vi "Actor Core.vi"(8 "error in":errorcluster, 11 "IMAQ Display in":refnum<class "HIJ Vision Display.lvclass">) -> (0 "error out":errorcluster, 3 "Actor out":refnum<class "Actor.lvclass">)   [LabVIEW 2020, in "HIJ Vision Display.lvlib" / "HIJ Vision Display.lvclass"]
doc: "(<B>Filename</B>: Actor Framework.lvlib:Actor.lvclass:Actor Core.vi)\n\nReceives messages to the actor, reacts to them, and initiates any error handling that may shut the actor down.\n\nDescendant classes may override this VI to append parallel tasks for the actor to complete while it handles messages. Overrides use the Call Parent Method node."
uses:
  HIJ Vision Display.lvclass
  C:/Users/AlexK/work/LabVIEW Programme/POLARIS CAM Log Abw und E/Submodules/Viewable Actor/ViewableActor/ViewableActor.lvclass
  C:/Program Files (x86)/National Instruments/LabVIEW 2020/vi.lib/ActorFramework/Actor/Actor.lvclass
  <vilib>/ActorFramework/Actor/Actor.lvclass
  Palette.ctl
  HIJ Vision Display.lvclass/HIJ Vision Display.ctl
  <vilib>/ActorFramework/Actor/Actor.lvclass/Actor.ctl
  <vilib>/ActorFramework/Message Enqueuer/Message Enqueuer.lvclass/Message Enqueuer.ctl
  HIJ Vision Display Messages/Write ROI Msg/Write ROI Msg.lvclass/Write ROI Msg.ctl
  HIJ Vision Display Messages/Mouse Click Coords Msg/Mouse Click Coords Msg.lvclass/Mouse Click Coords Msg.ctl
  HIJ Vision Display Messages/Send Reply Actor State/Send Reply Actor State.lvclass
  C:/Program Files (x86)/National Instruments/LabVIEW 2020/vi.lib/ActorFramework/Reply Msg/Reply Msg.lvclass
  <vilib>/ActorFramework/Message Enqueuer/Message Priority.ctl
  <vilib>/ActorFramework/Reply Msg/Reply Msg.lvclass/Reply Msg.ctl
  HIJ Vision Display Messages/Contex Menu Selection Msg/Contex Menu Selection Msg.lvclass/Contex Menu Selection Msg.ctl
  <vilib>/ActorFramework/Message Enqueuer/Init from Existing Queue.vi
  <vilib>/ActorFramework/Message Enqueuer/Enqueue.vi
  HIJ Vision Display Messages/Write ROI Msg/Write ROI Msg.lvclass
  C:/Program Files (x86)/National Instruments/LabVIEW 2020/vi.lib/ActorFramework/Message/Message.lvclass
  HIJ Vision Display Messages/Evaluate with new Params Msg/Evaluate with new Params Msg.lvclass
  HIJ Vision Display Messages/Mouse Click Coords Msg/Mouse Click Coords Msg.lvclass
  <vilib>/ActorFramework/Reply Msg/Reply Msg.lvclass
  HIJ Vision Display Messages/Contex Menu Selection Msg/Contex Menu Selection Msg.lvclass
  HIJ Vision Display Messages/Show or Hide QSettings Msg/Show or Hide QSettings Msg.lvclass
  <vilib>/ActorFramework/Message Priority Queue/Priority Enqueue.vi
  <vilib>/ActorFramework/Message Enqueuer/Message Enqueuer.lvclass
  Viewable Actor/ViewableActor/ViewableActor.lvclass
  Utility/POLARIS Vision utility.lvlib
  C:/Users/AlexK/work/LabVIEW Programme/POLARIS CAM Log Abw und E/Submodules/HIJ Vision/Display Actors/HIJ Vision Display/HIJ Vision Display Messages/Send Reply Actor State/Send Reply Actor State.lvclass
panel:
  out "Acq Stoped Ind":bool caption="Acquistion stoped!"
  in  "Zoom Buttons":T1(radio)
  out "Image":T2(plugin-control)
  in  "StopSignal":bool=TRUE
  in  "Pallete":T3={"Teiler"=1, "Palette Type"=2} {"Teiler" min=1 max=5; "Palette Type" items=["Grayscale", "Binary", "Gradient", "Rainbow", "Temperature", "User Defined"]}
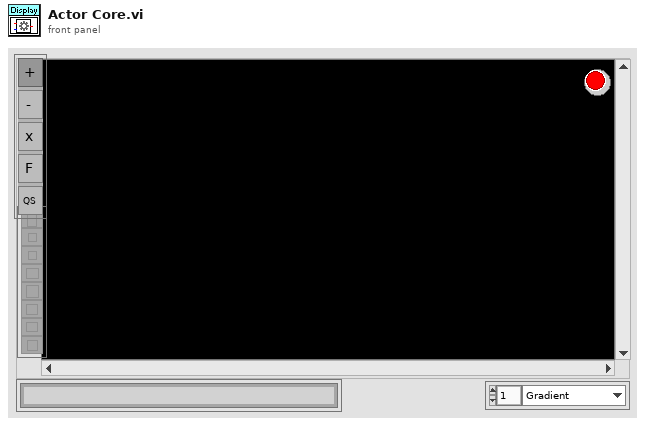
[diagram p1: front panel]
types:
  T1 = enum32{"Zoom in", "Zoom out", "Center", "Zoom to Fit", "Show Quick Settings"}
  T2 = typedef "IMAQ Image.ctl" = refnum<image>
  T3 = typedef "HIJ Vision Display.lvlib/HIJ Vision Display.lvclass/Palette.ctl" = cluster{"Teiler":i32, "Palette Type":u32}
  T4 = enum32{"Zoom in", "Zoom out", "Center", "Zoom to Fit"}
  T5 = cluster{"Zoom Tool":bool, "Selection Tool":bool, "Pan Tool":bool, "Point Tool":bool, "Line Tool":bool, "Rectangle Tool":bool, "Rotated Rectangle Tool":bool, "Polyline Tool":bool, "Polygon Tool":bool, "Freehand Tool":bool, "Closed Freehand Tool":bool, "Ellipse Tool":bool, "Annulus Tool":bool}
  T6 = typedef "Actor Framework.lvlib/Message Enqueuer.lvclass/Message Priority.ctl" = enum16{"Low", "Normal", "High"}
  T7 = cluster{"Global Rectangle":i32[], "Contours":cluster{"Contour Type":u32, "ROI Type":u32, "Points":i32[]}[]}
  T8 = typedef "LVPositionTypeDef.ctl" = cluster{"Left":i32, "Top":i32}
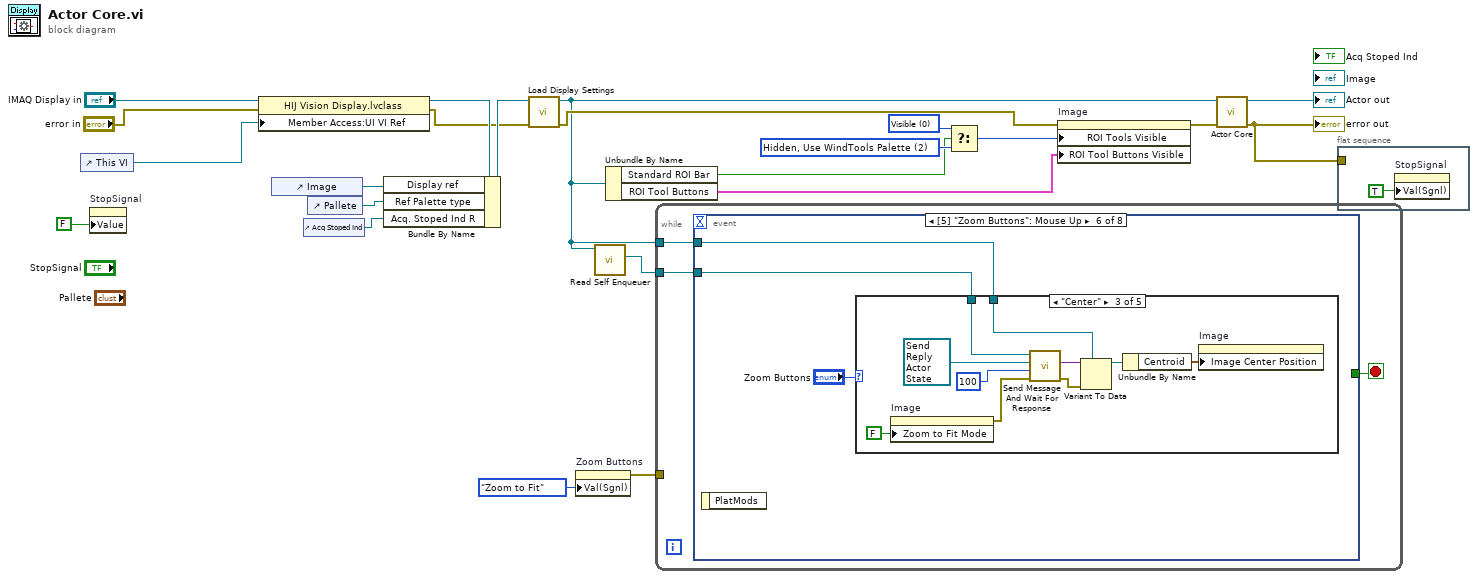
[diagram p0: block diagram]
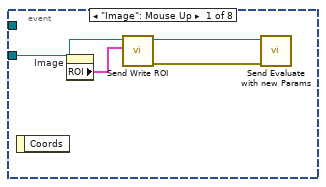
[diagram p2: hidden frame]
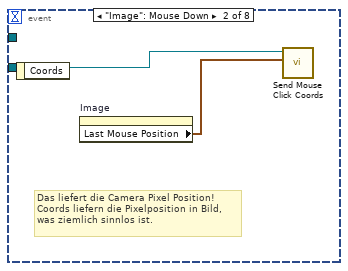
[diagram p3: hidden frame]
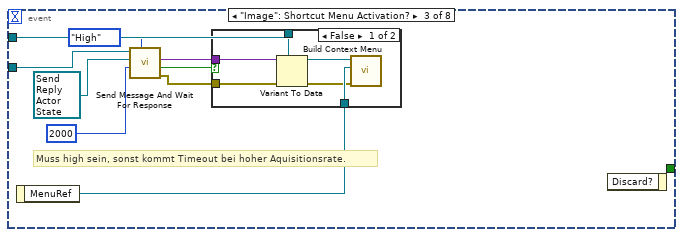
[diagram p4: hidden frame]
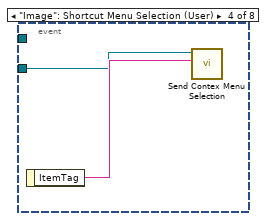
[diagram p6: hidden frame]
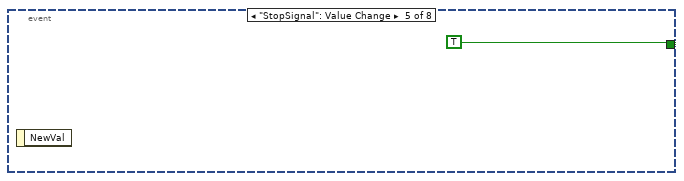
[diagram p7: hidden frame]
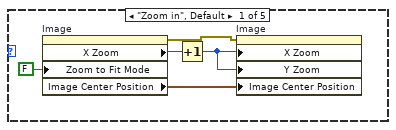
[diagram p8: hidden frame]
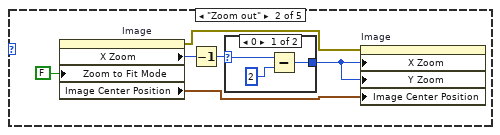
[diagram p9: hidden frame]
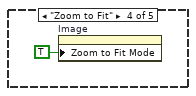
[diagram p11: hidden frame]
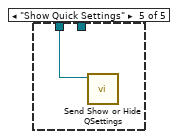
[diagram p12: hidden frame]
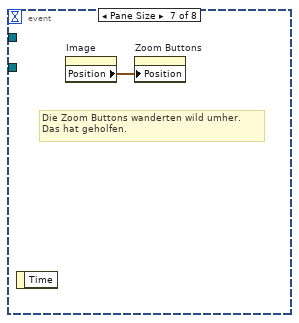
[diagram p13: hidden frame]
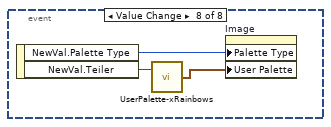
[diagram p14: hidden frame]
diagram:
  w3 = u32 0 items=["Visible", "Hidden", "Hidden, Use WindTools Palette"] ("ROI Tools Visible")
  w6 = u32 2 items=["Visible", "Hidden", "Hidden, Use WindTools Palette"] ("ROI Tools Visible")
  n1 = control-ref of="This VI"() -> (w16:refnum<vi>)
  n2 = property on="StopSignal" class="Bool (strict)"("Value"=FALSE ("Value (Signaling)")) -> ()  [unwired: 2 in, 2 out]
  n3 = property class="HIJ Vision Display.lvclass"(reference="IMAQ Display in", error in="error in", "Member Access:UI VI Ref"=w16) -> (reference out=w17:refnum<class "HIJ Vision Display.lvclass">, error out=w13:errorcluster)
  n4 = control-ref of="Image"() -> (w18:refnum<vi>)
  n5 = control-ref of="Acq Stoped Ind"() -> (w1:refnum<vi>)
  n6 = control-ref of="Pallete"() -> (w14:refnum<vi>)
  n7 = Bundle By Name(cluster=w17, "Display ref"=w18, "Ref Palette type"=w14, "Acq. Stoped Ind R"=w1) -> (w19:refnum<class "HIJ Vision Display.lvclass">)
  n8 = call-dynamic "Load Display Settings.vi"("error in (no error)"=w13, "AF IMAQ Display in"=w19) -> ("error out"=w12:errorcluster, "AF IMAQ Display out"=w8:refnum<class "HIJ Vision Display.lvclass">)  [unwired: 8 in]
  n9 = property on="Zoom Buttons" class="RadioBtnsControl (strict)"("Val(Sgnl)"=T4."Zoom to Fit" ("Value (Signaling)")) -> (error out=w9:errorcluster)  [unwired: 2 in, 1 out]
  n10 = call <vilib>:"Read Self Enqueuer.vi"("Actor"=w8) -> ("Self Enqueuer"=w11:refnum<class "Message Enqueuer.lvclass">)  [unwired: 10 in]
  n11 = Unbundle By Name(w8) -> ("Standard ROI Bar"=w4:bool, "ROI Tool Buttons"=w2:T5)
  n12 = while {
    tunnel: w11 -> [w26]
    tunnel: w8 -> [w25]
    tunnel: w9 -> [_]
    stop <- w24 stop-if-true
    n13 = event shown="[5] \"Zoom Buttons\": Mouse Up" {
      selector: _ -> [_ _ _ _ _ _ _ _]
      dyn-events: _ -> [_ _ _ _ _ _ _ _]
      timeout: _ -> [_ _ _ _ _ _ _ _]
      tunnel: w26 -> [w30 w32 w39 w48 _ w51 _ _]
      tunnel: w25 -> [_ _ w41 _ _ w52 _ _]
      tunnel: [_ _ _ _ TRUE _ _ _] -> w24
      event "Image": Mouse Up {
        n14 = event-data() -> ()  [unwired: 1 in, 1 out]
        n15 = property on="Image" class="ImageControl"() -> ("ROI"=w29:T7)  [unwired: 2 in, 2 out]
        n16 = call "Send Write ROI.vi"("ROI Descriptor"=w29, "Message Enqueuer"=w30) -> ("error out"=w27:errorcluster, "Message Enqueuer out"=w28:refnum<class "Message Enqueuer.lvclass">)  [unwired: 8 in]
        n17 = call "Send Evaluate with new Params.vi"("error in (no error)"=w27, "Message Enqueuer"=w28) -> ()  [unwired: 8 in, 2 out]
      }
      event "Image": Mouse Down {
        # "Das liefert die Camera Pixel Position!\nCoords liefern die Pixelposition in Bild,\nwas ziemlich sinnlos ist."
        n18 = event-data() -> ()  [unwired: 1 in, 1 out]
        n19 = property on="Image" class="ImageControl"() -> ("Last Mouse Position"=w31:cluster{"X":i32, "Y":i32})  [unwired: 2 in, 2 out]
        n20 = call "Send Mouse Click Coords.vi"("Coords"=w31, "Message Enqueuer"=w32) -> ()  [unwired: 8 in, 2 out]
      }
      event "Image": Shortcut Menu Activation? {
        # "Muss high sein, sonst kommt Timeout bei hoher Aquisitionsrate."
        n21 = event-data() -> ("MenuRef"=w40:refnum<k9>)  [unwired: 1 in]
        n22 = call <vilib>:"Send Message And Wait For Response.vi"("Message Priority (Normal)"=Message_Priority."High", "timeout in ms (-1)"=2000, "Original Message"=refnum<class "Send Reply Actor State.lvclass"> refnum ("IMAQ Display.lvlib:Send Reply Actor State.lvclass"), "Message Enqueuer in"=w39) -> ("error out"=w38:errorcluster, "timed out?"=w34:bool, "Reply"=w37:variant)  [unwired: 4 in, 1 out]
        n23 = case shown="False" w34 {
          tunnel: w38 -> [w47 _]
          tunnel: w37 -> [w46 _]
          tunnel: w41 -> [w45 _]
          tunnel: w40 -> [w44 _]
          frame False {
            n24 = Variant To Data(error in=w47, type=w45, Variant=w46) -> (data=w42:refnum<class "HIJ Vision Display.lvclass">, error out=w43:errorcluster)
            n25 = call-dynamic "Build Context Menu.vi"("error in (no error)"=w43, "MenuRef"=w44, "HIJ Vision Display in"=w42) -> ()  [unwired: 6 in, 3 out]
          }
          frame True {
          }
        }
        n26 = event-data() -> ()  [unwired: 2 in, 1 out]
      }
      event "Image": Shortcut Menu Selection (User) {
        n27 = event-data() -> ("ItemTag"=w49:string)  [unwired: 1 in]
        n28 = call "Send Contex Menu Selection.vi"("MenuItem"=w49, "Message Enqueuer"=w48) -> ()  [unwired: 8 in, 2 out]
      }
      event "StopSignal": Value Change {
        n29 = event-data() -> ()  [unwired: 1 in, 1 out]
      }
      event "Zoom Buttons": Mouse Up {
        n30 = event-data() -> ()  [unwired: 1 in, 1 out]
        n31 = case shown="\"Center\"" "Zoom Buttons" {
          tunnel: w52 -> [_ _ w78 _ _]
          tunnel: w51 -> [_ _ w72 _ w80]
          frame "Zoom in", Default {
            n32 = property on="Image" class="ImageControl"("Zoom to Fit Mode"=FALSE) -> (error out=w56:errorcluster, "X Zoom"=w57:i32, "Image Center Position"=w58:cluster{"X":u32, "Y":u32})  [unwired: 2 in, 1 out]
            n33 = Increment(x=w57) -> (x+1=w55:i32)
            n34 = property on="Image" class="ImageControl"(error in=w56, "X Zoom"=w55, "Y Zoom"=w55, "Image Center Position"=w58) -> ()  [unwired: 1 in, 2 out]
          }
          frame "Zoom out" {
            n35 = property on="Image" class="ImageControl"("Zoom to Fit Mode"=FALSE) -> (error out=w61:errorcluster, "X Zoom"=w63:i32, "Image Center Position"=w62:cluster{"X":u32, "Y":u32})  [unwired: 2 in, 1 out]
            n36 = Decrement(x=w63) -> (x-1=w64:i32)
            n37 = case shown="0" w64 {
              selector: w64 -> [w67 w68]
              tunnel: [w66 w68] -> w60
              frame 0 {
                n38 = Subtract(x=w67, y=2 ("x")) -> (x-y=w66:i32)
              }
              frame 1, Default {
              }
            }
            n39 = property on="Image" class="ImageControl"(error in=w61, "X Zoom"=w60, "Y Zoom"=w60, "Image Center Position"=w62) -> ()  [unwired: 1 in, 2 out]
          }
          frame "Center" {
            n40 = property on="Image" class="ImageControl"("Zoom to Fit Mode"=FALSE) -> (error out=w70:errorcluster)  [unwired: 2 in, 1 out]
            n41 = call <vilib>:"Send Message And Wait For Response.vi"("error in (no error)"=w70, "timeout in ms (-1)"=100, "Original Message"=refnum<class "Send Reply Actor State.lvclass"> refnum ("IMAQ Display.lvlib:Send Reply Actor State.lvclass"), "Message Enqueuer in"=w72) -> ("error out"=w73:errorcluster, "Reply"=w74:variant)  [unwired: 4 in, 2 out]
            n42 = Variant To Data(error in=w73, type=w78, Variant=w74) -> (data=w69:refnum<class "HIJ Vision Display.lvclass">)  [unwired: 1 out]
            n43 = Unbundle By Name(w69) -> ("Centroid"=w77:cluster{"X Centroid":sgl, "Y Centroid":sgl})
            n44 = property on="Image" class="ImageControl"("Image Center Position"=w77) -> ()  [unwired: 2 in, 2 out]
          }
          frame "Zoom to Fit" {
            n45 = property on="Image" class="ImageControl"("Zoom to Fit Mode"=TRUE) -> ()  [unwired: 2 in, 2 out]
          }
          frame "Show Quick Settings" {
            n46 = call "Send Show or Hide QSettings.vi"("Message Enqueuer"=w80) -> ()  [unwired: 9 in, 2 out]
          }
        }
      }
      event Pane Size {
        # "Die Zoom Buttons wanderten wild umher.\nDas hat geholfen."
        n47 = event-data() -> ()  [unwired: 1 in, 1 out]
        n48 = property on="Image" class="ImageControl"() -> ("Position"=w81:T8)  [unwired: 2 in, 2 out]
        n49 = property on="Zoom Buttons" class="RadioBtnsControl (strict)"("Position"=w81) -> ()  [unwired: 2 in, 2 out]
      }
      event Value Change {
        n50 = event-data() -> ("NewVal.Palette Type"=w83:u32, "NewVal.Teiler"=w84:i32)  [unwired: 1 in]
        n51 = call "UserPalette-xRainbows.vi"("Teiler"=w84) -> ("Array"=w82:cluster{u8, u8, u8}[])  [unwired: 1 in]
        n52 = property on="Image" class="ImageControl"("Palette Type"=w83, "User Palette"=w82) -> ()  [unwired: 2 in, 2 out]
      }
    }
  }
  n53 = Select(t=w3, s=w4, f=w6) -> (s? t:f=w5:u32)
  n54 = property on="Image" class="ImageControl"(error in=w12, "ROI Tools Visible"=w5, "ROI Tool Buttons Visible"=w2) -> (error out=w7:errorcluster)  [unwired: 1 in, 1 out]
  n55 = call-parent "Actor Core.vi"("error in"=w7, "Actor in"=w8) -> ("error out"=w21:errorcluster, "Actor out"=→"Actor out":refnum<class "Actor.lvclass">)  [unwired: 8 in]
  "error out" <- w21
  n56 = flat-sequence {
    tunnel: w21 -> [_]
    frame #0 {
      n57 = property on="StopSignal" class="Bool (strict)"("Val(Sgnl)"=TRUE ("Value (Signaling)")) -> ()  [unwired: 2 in, 2 out]
    }
  }
